vi "Check String.vi"(0 "Data Length":i32, 2 "Measurement":string, 3 "Expression":string) -> (1 "Data Out":string)   [LabVIEW 2023]
uses:
  <vilib>/regexp/Match Regular Expression.xnode
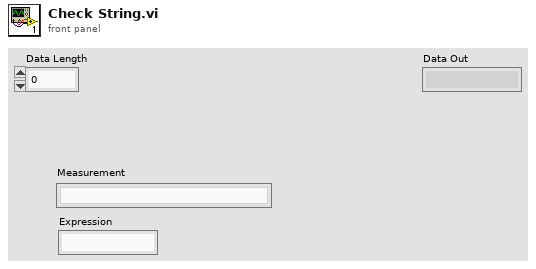
[diagram p1: front panel]
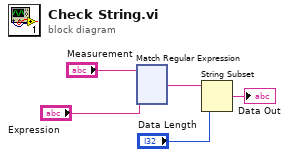
[diagram p0: block diagram]
diagram:
  n1 = xnode "Match Regular Expression"("input string"="Measurement", "regular expression"="Expression") -> ("after match"=w4:string)  [unwired: 4 in, 4 out]
  n2 = String Subset(string=w4, length (rest)="Data Length") -> (substring=→"Data Out":string)  [unwired: 1 in]
